vi "PulseblasterLabviewLoad_MR1.vi"(2 "error in (no error)":errorcluster, 3 "Input file":path=path "C:/Users/Lab/Desktop/Pulseblaster Interpreter Codes/channel_selectMR1.pb") -> (0 "error out":errorcluster, 1 "standard output":string="Labels:\r\nLABEL = 1\r\n\r\nVariables:\r\n\r\nProgram Lines:\r\nLine 1: 0B000000000000111100000000, 500MS, CONTINUE, 0\r\nLine 2: 0B000000100000000000001110, 1S, CONTINUE, 0\r\nLine 3: 0B000000100000000000001110, 1S, BRANCH, LABEL\r\n\r\nUsing Clock Frequency of 100 MHz.\r\n\r\nParse Values:\r\nLine 1: 3840 5e+08 0 0\r\nLine 2: 131086 1e+09 0 0\r\nLine 3: 131086 1e+09 6 1\r\n\r\n3 instructions interpreted.\r\nBoard programmed successfully.\r\n")   [LabVIEW 2016]
panel:
  out "Full command to cmd":string="cmd /c spbicl load \"C:\\Users\\Lab\\Desktop\\Pulseblaster Interpreter Codes\\channel_selectMR1.pb\" 100.0"
  out "standard error":string
  out "return code":i32
  in  "Pulseblaster interpreter directory":path=path "C:/SpinCore/SpinAPI/interpreter"
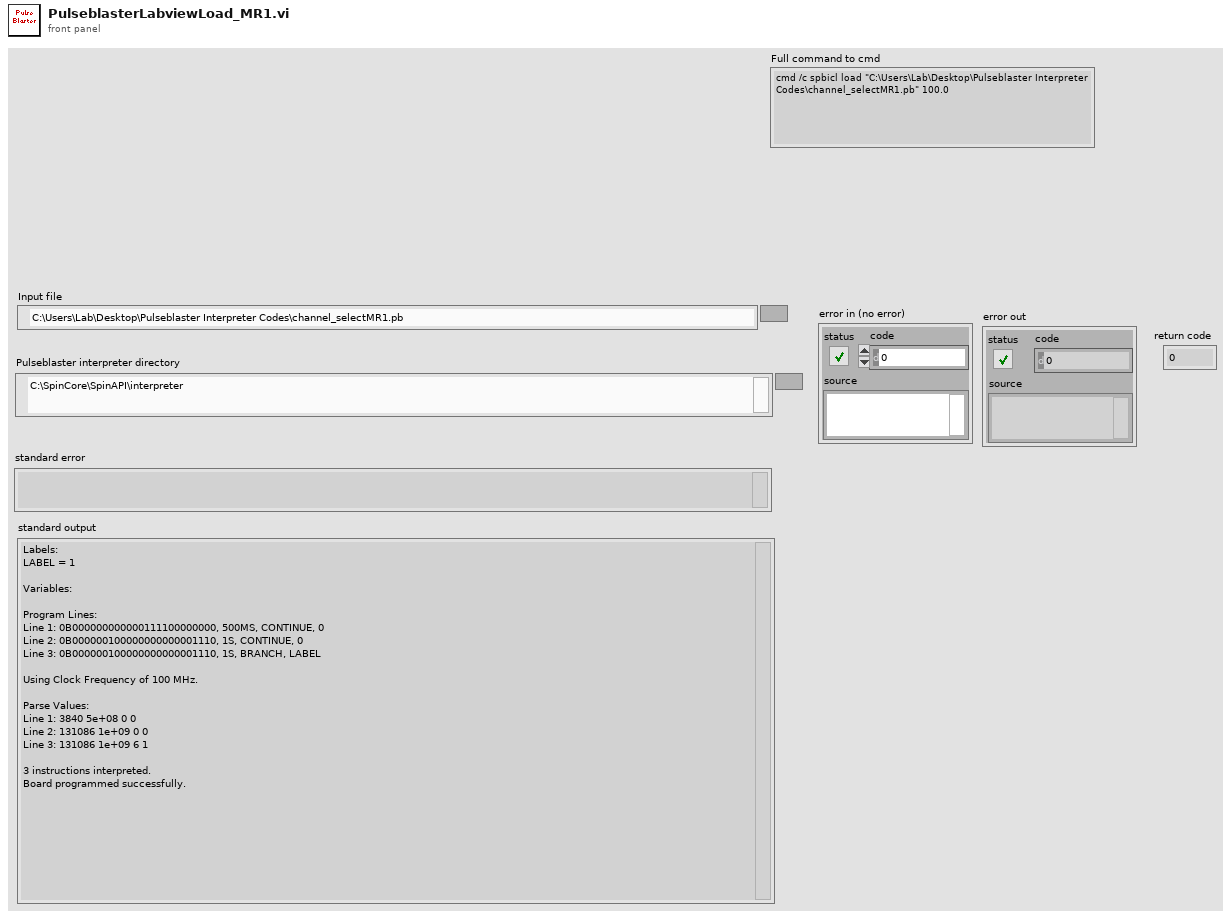
[diagram p1: front panel]
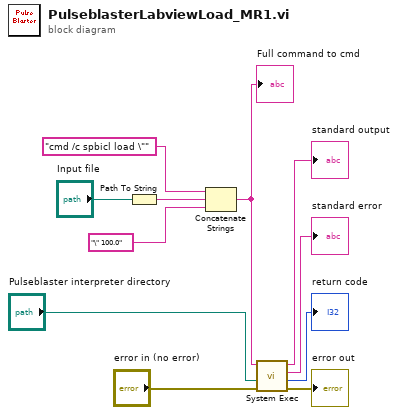
[diagram p0: block diagram]
diagram:
  n1 = Path To String(path="Input file") -> (string=w1:string)
  n2 = Concatenate Strings("cmd /c spbicl load \"" ("string"), w1, "\" 100.0" ("string")) -> (w3:string)
  "Full command to cmd" <- w3
  n3 = call <vilib>:"System Exec.vi"("error in (no error)"="error in (no error)", "working directory"="Pulseblaster interpreter directory", "command line"=w3) -> ("error out"=→"error out":errorcluster, "return code"=→"return code":i32, "standard error"=→"standard error":string, "standard output"=→"standard output":string)  [unwired: 5 in]
